vi "Read Obstacle File.vi"(8 "error in (no error)":errorcluster, 10 "file path (use dialog)":path) -> (0 "error out":errorcluster, 2 "obstacles (n x 2 array of pts)":cluster{dbl, dbl}[][](array[cluster]))   [LabVIEW 2011]
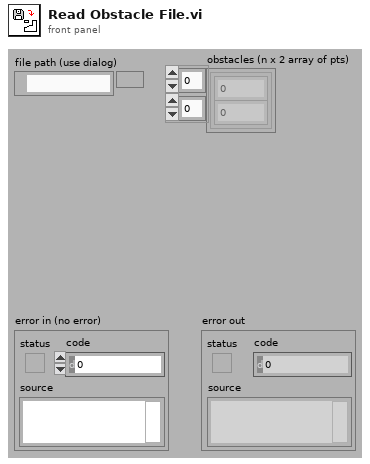
[diagram p1: front panel]
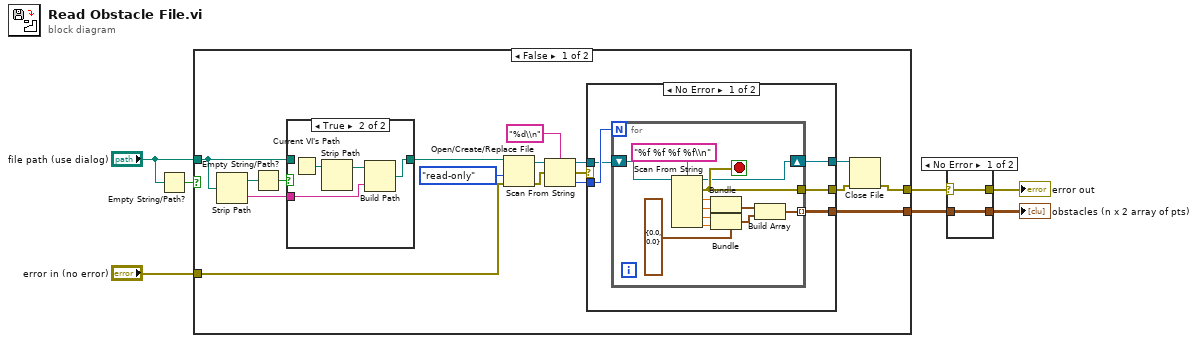
[diagram p0: block diagram]
diagram:
  n1 = Empty String/Path?(string/path="file path (use dialog)") -> (empty?=w6:bool)
  n2 = case shown="False" w6 {
    tunnel: [w19 _] -> w5
    tunnel: [w14 w49] -> w2
    tunnel: "file path (use dialog)" -> [w11 _]
    tunnel: "error in (no error)" -> [w8 w49]
    frame False {
      n3 = Strip Path(path=w11) -> (stripped path=w13:path, name=w12:string)
      n4 = Empty String/Path?(string/path=w13) -> (empty?=w10:bool)
      n5 = case shown="True" w10 {
        tunnel: w12 -> [_ w27]
        tunnel: w11 -> [w25 _]
        tunnel: [w25 w26] -> w9
        frame False {
        }
        frame True {
          n6 = Current VI's Path() -> (path=w29:path)
          n7 = Strip Path(path=w29) -> (stripped path=w28:path)  [unwired: 1 out]
          n8 = Build Path(base path=w28, name or relative path=w27) -> (appended path=w26:path)
        }
      }
      n9 = Open/Create/Replace File(file path (use dialog)=w9, error in=w8, access (0:read/write)=enum16{"read/write", "read-only", "write-only"}."read-only") -> (refnum out=w23:refnum<file>, error out=w18:errorcluster)  [unwired: 4 out]
      n10 = Scan From String("%d\\n" ("format string"), w23, w18) -> (w17:refnum<file>, w20:errorcluster, output 1=w21:i32)  [unwired: 1 out]
      n11 = case shown="No Error" w20 {
        selector: w20 -> [_ w48]
        tunnel: w21 -> [w34 _]
        tunnel: [w33 w48] -> w16
        tunnel: [w32 _] -> w19
        tunnel: w17 -> [w31 w47]
        tunnel: [w30 w47] -> w15
        frame No Error {
          n12 = for {
            N: w34 -> [_]
            tunnel: [w45] -> w33
            tunnel: [w37] -> w32 mode=indexing
            shift-right: [w35] -> w30
            shift-left: w31 -> [w36]
            stop <- w45 stop-if-true
            w44 = cluster{"X":dbl, "Y":dbl} {"X"=0.0, "Y"=0.0}
            n13 = Scan From String("%f %f %f %f\\n" ("format string"), w36) -> (w35:refnum<file>, w45:errorcluster, output 1=w43:dbl, output 2=w42:dbl, output 3=w41:dbl, output 4=w40:dbl)  [unwired: 1 in, 4 out]
            n14 = Bundle(cluster=w44, "X"=w43, "Y"=w42) -> (w38:cluster{"X":dbl, "Y":dbl})
            n15 = Bundle(cluster=w44, "X"=w41, "Y"=w40) -> (w39:cluster{"X":dbl, "Y":dbl})
            n16 = Build Array(w38, w39) -> (w37:cluster{"X":dbl, "Y":dbl}[])
          }
        }
        frame Error {
        }
      }
      n17 = Close File(refnum=w15, error in=w16) -> (error out=w14:errorcluster)  [unwired: 1 out]
    }
    frame True {
    }
  }
  n18 = case shown="No Error" w2 {
    selector: w2 -> [w50 w52]
    tunnel: w5 -> [w51 _]
    tunnel: [w51 _] -> w4
    tunnel: [w50 w52] -> w1
    frame No Error {
    }
    frame Error {
    }
  }
  "obstacles (n x 2 array of pts)" <- w4
  "error out" <- w1
